vi "Initialize EtherCAT youBot Arm Motor.vi"(8 "error in (no error)":errorcluster, 9 "arm motor param":T1={"ticks per radian"=1.0, "ticks offset"=0, "calibration max current (A)"=1.0, "torqure constant (Nm/A)"=0.0, "do calibration?"=FALSE, "positive calibtration direction?"=FALSE}, 11 "motor slave info in":T2 {"nodeAddr" format="%.0x"}) -> (0 "error out":errorcluster, 3 "KUKA youBot arm motor_EtherCAT out":refnum<class "NI_Robotics_KUKA youBot Arm Motor_EtherCAT.lvclass">)   [LabVIEW 2017, in "NI_Robotics_KUKA youBot Host.lvlib" / "NI_Robotics_KUKA youBot Arm Motor_EtherCAT.lvclass"]
uses:
  <vilib>/robotics/KUKA youBot/Motor/Arm Motor EtherCAT/NI_Robotics_KUKA youBot Arm Motor_EtherCAT.lvclass
  <vilib>/robotics/KUKA youBot/EtherCAT/Motor Slave Info.ctl
  <vilib>/robotics/KUKA youBot/EtherCAT/LowLevel/Mater Handler.ctl
  <vilib>/robotics/KUKA youBot/Motor/Arm Motor EtherCAT/Arm Motor Parameter.ctl
  <vilib>/robotics/KUKA youBot/EtherCAT/EtherCAT Command.ctl
  <vilib>/robotics/KUKA youBot/EtherCAT/CmdCtrls/Param Cmd.ctl
  <vilib>/robotics/KUKA youBot/Motor/Arm Motor EtherCAT/NI_Robotics_KUKA youBot Arm Motor_EtherCAT.lvclass/NI_Robotics_KUKA youBot Arm Motor_EtherCAT.ctl
  <vilib>/robotics/KUKA youBot/NI_Robotics_KUKA youBot Host.lvlib
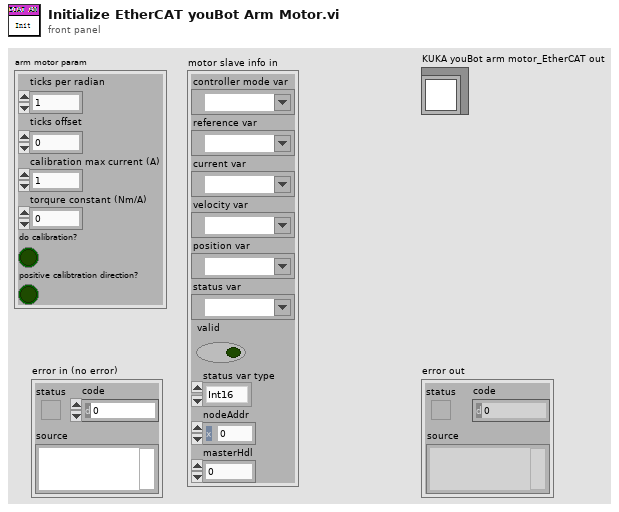
[diagram p1: front panel]
types:
  T1 = typedef "NI_Robotics_KUKA youBot Host.lvlib/NI_Robotics_KUKA youBot Arm Motor_EtherCAT.lvclass/Arm Motor Parameter.ctl" = cluster{"ticks per radian":dbl, "ticks offset":i32, "calibration max current (A)":dbl, "torqure constant (Nm/A)":dbl, "do calibration?":bool, "positive calibtration direction?":bool}
  T2 = typedef "NI_Robotics_KUKA youBot Host.lvlib/Motor Slave Info.ctl" = cluster{"controller mode var":refnum<k21>, "reference var":refnum<k21>, "current var":refnum<k21>, "velocity var":refnum<k21>, "position var":refnum<k21>, "status var":refnum<k21>, "valid":bool, "status var type":enum16{"Int16", "Int32"}, "nodeAddr":u16, "masterHdl":T3}
  T3 = typedef "NI_Robotics_KUKA youBot Host.lvlib/Mater Handler.ctl" = i32
  T4 = typedef "NI_Robotics_KUKA youBot Host.lvlib/EtherCAT Command.ctl" = cluster{"Module":u8, "Cmd":T5, "Type":u8, "Bank":u8, "Val":u32}
  T5 = typedef "NI_Robotics_KUKA youBot Host.lvlib/Param Cmd.ctl" = u8
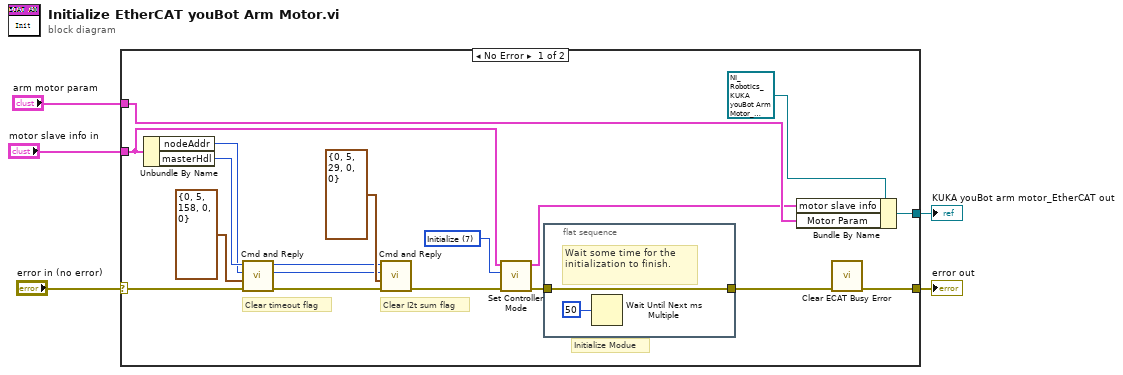
[diagram p0: block diagram]
diagram:
  n1 = case shown="No Error" "error in (no error)" {
    selector: "error in (no error)" -> [w16 w26]
    tunnel: [w10 w26] -> w4
    tunnel: [w23 _] -> w2
    tunnel: "motor slave info in" -> [w19 _]
    tunnel: "arm motor param" -> [w20 _]
    frame No Error {
      w21 = u8 7 items=["Motor Stop", "Positioning-Mode", "Velocity-Mode", "no more action", "set position to reference", "PWM-Mode", "Current-Mode", "Initialize"] ("controller mode")
      # "Clear I2t sum flag"
      # "Clear timeout flag"
      # "Initialize Modue"
      n2 = Unbundle By Name(w19) -> ("nodeAddr"=w12:u16, "masterHdl"=w15:T3)
      n3 = call <vilib>:"Cmd and Reply.vi"("error in (no error)"=w16, "EtherCAT command"=T4 {"Module"=0, "Cmd"=5, "Type"=158, "Bank"=0, "Val"=0} ("EtherCAT Command"), "nodeAddr in"=w12, "masterHdl in"=w15) -> ("error out"=w7:errorcluster, "nodeAddr out"=w13:u16, "masterHdl out"=w14:T3)  [unwired: 3 in, 2 out]
      n4 = call <vilib>:"Cmd and Reply.vi"("error in (no error)"=w7, "EtherCAT command"=T4 {"Module"=0, "Cmd"=5, "Type"=29, "Bank"=0, "Val"=0} ("EtherCAT Command"), "nodeAddr in"=w13, "masterHdl in"=w14) -> ("error out"=w6:errorcluster)  [unwired: 3 in, 4 out]
      n5 = call <vilib>:"Set Controller Mode.vi"("error in (no error)"=w6, "controller mode"=w21, "motor slave info in"=w19) -> ("error out"=w18:errorcluster, "motor slave info out"=w8:T2)  [unwired: 6 in, 1 out]
      n6 = flat-sequence {
        tunnel: w18 -> [w24]
        tunnel: [w24] -> w9
        frame #0 {
          # "Wait some time for the initialization to finish."
          n7 = Wait Until Next ms Multiple(millisecond multiple=u32 50) -> ()  [unwired: 1 out]
        }
      }
      n8 = Bundle By Name(cluster=refnum<class "NI_Robotics_KUKA youBot Arm Motor_EtherCAT.lvclass"> refnum ("NI_Robotics_KUKA youBot Host.lvlib:NI_Robotics_KUKA youBot Arm Motor_EtherCAT.lvclass"), "motor slave info"=w8, "Motor Param"=w20) -> (w23:refnum<class "NI_Robotics_KUKA youBot Arm Motor_EtherCAT.lvclass">)
      n9 = call <vilib>:"Clear ECAT Busy Error.vi"("error in (no error)"=w9) -> ("error out"=w10:errorcluster)  [unwired: 10 in]
    }
    frame Error {
    }
  }
  "error out" <- w4
  "KUKA youBot arm motor_EtherCAT out" <- w2
